vi "Write Channels_ AO.vi"(8 "error in (no error)":errorcluster, 10 "Channels: AO":T1={"Ch"=[], "Amp (V)"=[0.01, 0.0, 0.0, 0.0, 0.0, 0.0, 0.0, 0.0], "DC (V)"=[0.0, 0.0, 0.0, 0.0, 0.0, 0.0, 0.0, 0.0], "f (Hz)"=[0.0, 0.0, 0.0, 0.0, 0.0, 0.0, 0.0, 0.0], "Phase (°)"=[13.1, 13.0, 13.0, 13.0, 13.0, 13.0, 13.0, 13.0], "Function"=[enum."Sine", enum."Sine", enum."Sine", enum."Sine", enum."Sine", enum."Sine", enum."Sine", enum."Sine"], "Sweep?"=[FALSE, FALSE, FALSE, FALSE, FALSE, FALSE, FALSE, FALSE]} {"f (Hz)" min=0.001 max=10000.0 format="%.3g"; "Phase (°)" format="%.3g"; "DC (V)" format="%.3p"; "Amp (V)" min=0.0 max=10.0 format="%.3p"}, 11 "LockinDAQ":refnum<class "LockinDAQ.lvclass">) -> (0 "error out":errorcluster, 3 "LockinDAQ out":refnum<class "LockinDAQ.lvclass">)   [LabVIEW 2016, in "LockinDAQ.lvclass"]
uses:
  LockinDAQ.lvclass
  Typedefs/AO-cluster.ctl
  Typedefs/Function-enum.ctl
  LockinDAQ.lvclass/LockinDAQ.ctl
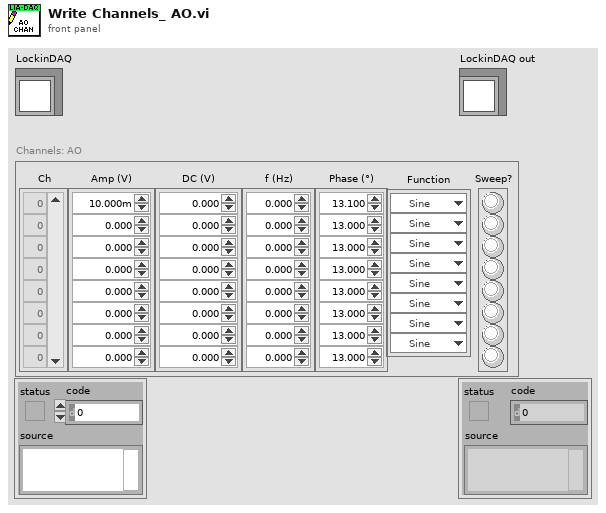
[diagram p1: front panel]
types:
  T1 = typedef "LockinDAQ.lvclass/AO-cluster.ctl" = cluster{"Ch":i32[], "Amp (V)":dbl[], "DC (V)":dbl[], "f (Hz)":dbl[], "Phase (°)":dbl[], "Function":T2[], "Sweep?":bool[]}
  T2 = typedef "LockinDAQ.lvclass/Function-enum.ctl" = enum16{"Sine", "Triangle", "Square", "Sawtooth"}
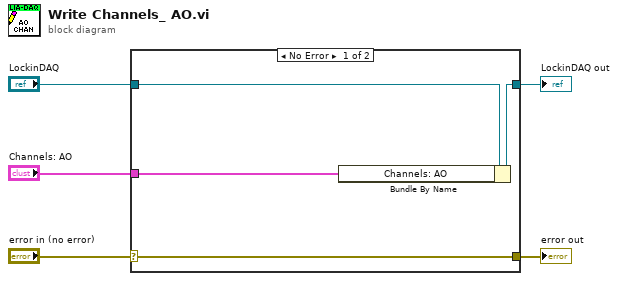
[diagram p0: block diagram]
diagram:
  n1 = case shown="No Error" "error in (no error)" {
    selector: "error in (no error)" -> [w9 w10]
    tunnel: [w9 w10] -> w4
    tunnel: [w7 w11] -> w2
    tunnel: "LockinDAQ" -> [w8 w11]
    tunnel: "Channels: AO" -> [w6 _]
    frame No Error {
      n2 = Bundle By Name(cluster=w8, "Channels: AO"=w6) -> (w7:refnum<class "LockinDAQ.lvclass">)
    }
    frame Error {
    }
  }
  "error out" <- w4
  "LockinDAQ out" <- w2
